vi "Unit Discrete Delay (Boolean).vi"(7 "Input":bool) -> (8 "Output":bool)   [LabVIEW 2011]
uses:
  <vilib>/rvi/FXPMathLib/basic elements/FxpDiscreteDelay/XNode/nifxpmath_DiscreteDelay.xnode
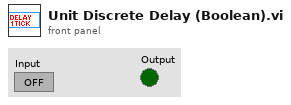
[diagram p1: front panel]
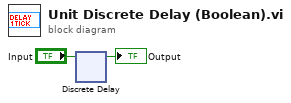
[diagram p0: block diagram]
diagram:
  n1 = xnode "Discrete Delay"("D"="Input") -> ("Q"=→"Output":bool)
